vi "lab session 2.1V.vi"(1 "deg C":dbl) -> (0 "deg F":dbl)   [LabVIEW 2020]
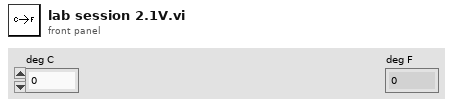
[diagram p1: front panel]
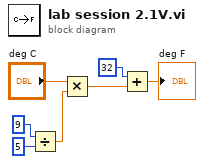
[diagram p0: block diagram]
diagram:
  n1 = Divide(x=9, y=5) -> (x/y=w5:dbl)
  n2 = Multiply(x="deg C", y=w5) -> (x*y=w3:dbl)
  n3 = Add(x=32, y=w3) -> (x+y=→"deg F":dbl)
